vi "Initialize Scanning Task.vi"(0 "NI Force Task in":refnum<class "NI Force Task.lvclass">, 1 "Pot Calibration Cluster":cluster{"Left":dbl, "Right":dbl}, 2 "TDMS File":refnum<k34>, 3 "EMG info":cluster{"Collect EMG?":bool, "EMG Rate":u16}, 4 "DAQ  Channels In":T1={"Force Transducer: Left"="Dev1/ai6", "Force Transducer: Right "="Dev1/ai8", "EMG: Left"="", "EMG: Right"="", "Potentiometer: Left"="", "Potentiometer: Right"=""}, 5 "error in (no error)":errorcluster, 7 "Task Info In":T2={"Number of Trials"=1, "Sampling Rate (Hz)"=200, "Trial Duration (s)"=10, "Adjusted MVC (N)"=5.0, "R Phase"=0, "L Phase"=0, "L Pattern"=1, "R Pattern"=1, "Time Between Trials (s)"=5, "Lissajous Speed"=200} {"Lissajous Speed" min=1 max=200; "Time Between Trials (s)" min=1 step=1; "R Pattern" min=1 max=20 step=1; "L Pattern" min=1 max=20 step=1; "L Phase" max=360 step=1; "R Phase" max=360 step=1; "Adjusted MVC (N)" min=1.0 step=1.0; "Trial Duration (s)" min=1 step=1; "Sampling Rate (Hz)" min=1 step=1; "Number of Trials" min=1 step=1}) -> (14 "NI Force Task out":refnum<class "NI Force Task.lvclass">, 19 "error out":errorcluster)   [LabVIEW 2020, in "NI Force Task.lvlib" / "NI Force Task.lvclass"]
uses:
  NI Force Task.lvclass
  Task info df.ctl
  NI Force Task.lvclass/NI Force Task.ctl
  <vilib>/DAQmx/create/channels.llb/DAQmx Create Channel (AI-Voltage-Basic).vi
  <vilib>/DAQmx/configure/timing.llb/DAQmx Timing (Sample Clock).vi
panel:
  out "error out 2":errorcluster
  # "Left Arm"
  # "Right Arm"
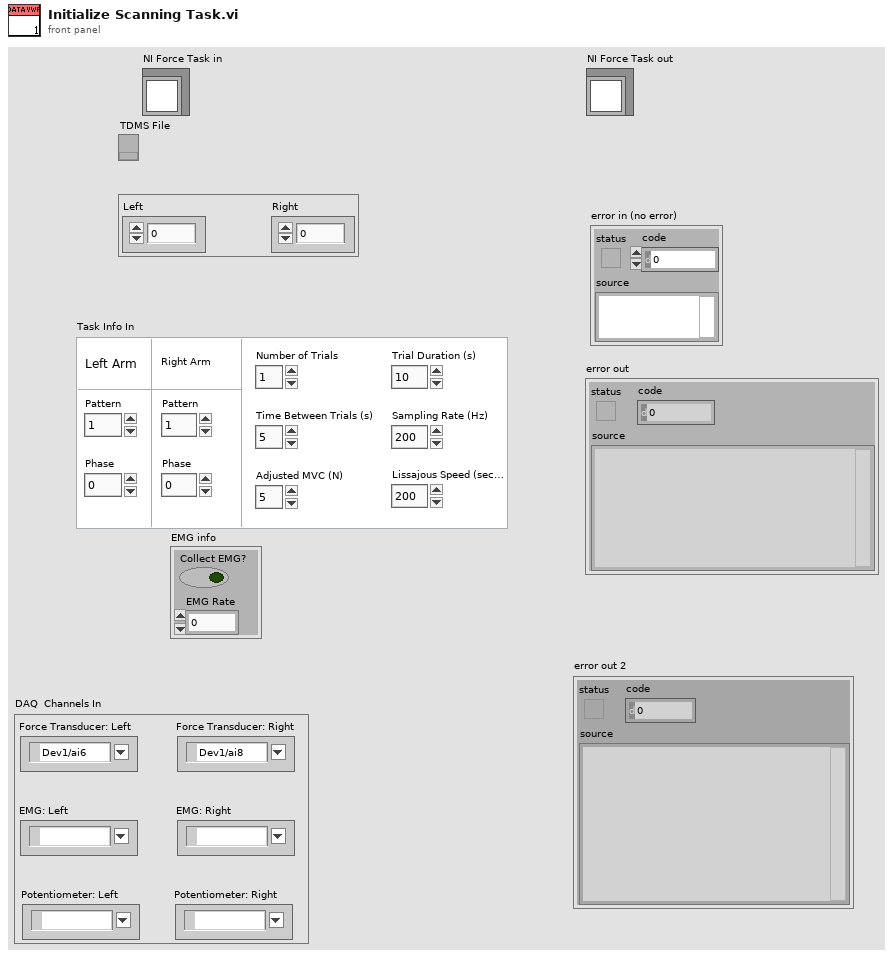
[diagram p1: front panel]
types:
  T1 = cluster{"Force Transducer: Left":tag, "Force Transducer: Right ":tag, "EMG: Left":tag, "EMG: Right":tag, "Potentiometer: Left":tag, "Potentiometer: Right":tag}
  T2 = typedef "Task info df.ctl" = cluster{"Number of Trials":u8, "Sampling Rate (Hz)":u16, "Trial Duration (s)":u8, "Adjusted MVC (N)":dbl, "R Phase":i32, "L Phase":i32, "L Pattern":u8, "R Pattern":u8, "Time Between Trials (s)":u8, "Lissajous Speed":u16}
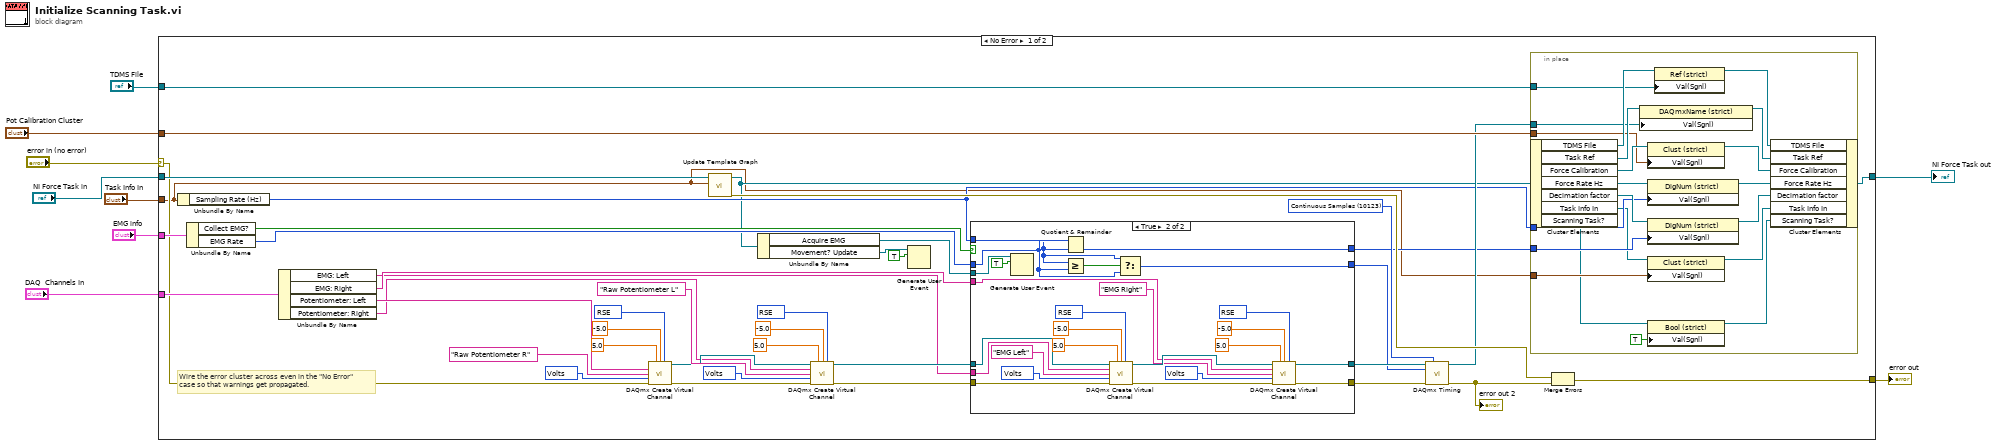
[diagram p0: block diagram]
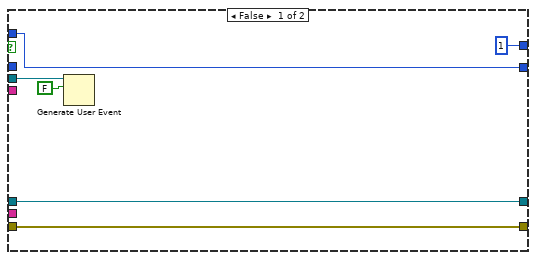
[diagram p2: hidden frame]
diagram:
  n1 = case shown="No Error" "error in (no error)" {
    selector: "error in (no error)" -> [w27 w105]
    tunnel: [w24 w105] -> w8
    tunnel: [w23 w104] -> w6
    tunnel: "NI Force Task in" -> [w51 w104]
    tunnel: "Task Info In" -> [w10 _]
    tunnel: "EMG info" -> [w50 _]
    tunnel: "DAQ  Channels In" -> [w48 _]
    tunnel: "Pot Calibration Cluster" -> [w22 _]
    tunnel: "TDMS File" -> [w20 _]
    frame No Error {
      w28 = 10123 items=["Finite Samples"=10178, "Continuous Samples"=10123, "Hardware Timed Single Point"=12522] ("sample mode")
      w38 = 10348 items=["Volts"=10348, "From Custom Scale"=10065] ("units")
      w42 = 10083 items=["Default"=-1, "RSE"=10083, "NRSE"=10078, "Differential"=10106, "Pseudodifferential"=12529] ("input terminal configuration")
      w43 = 10348 items=["Volts"=10348, "From Custom Scale"=10065] ("units")
      w47 = 10083 items=["Default"=-1, "RSE"=10083, "NRSE"=10078, "Differential"=10106, "Pseudodifferential"=12529] ("input terminal configuration")
      # "Wire the error cluster across even in the \"No Error\"\ncase so that warnings get propagated."
      n2 = Unbundle By Name(w10) -> ("Sampling Rate (Hz)"=w15:u16)
      n3 = Unbundle By Name(w50) -> ("Collect EMG?"=w49:bool, "EMG Rate"=w29:u16)
      n4 = Unbundle By Name(w48) -> ("EMG: Left"=w17:tag, "EMG: Right"=w18:tag, "Potentiometer: Left"=w35:tag, "Potentiometer: Right"=w34:tag)
      n5 = call-poly <vilib>:"DAQmx Create Virtual Channel.vi"("maximum value"=5.0, "minimum value"=-5.0, "input terminal configuration"=w47, "physical channels"=w35, "name to assign"="Raw Potentiometer R", "units"=w43, "error in"=w27) -> ("task out"=w37:refnum<k21>, "error out"=w36:errorcluster)  [unwired: 7 in]
      n6 = call "Update Template Graph.vi"("Task Info In"=w10, "NI Force Task in"=w51) -> ("error out"=w26:errorcluster, "NI Force Task out"=w14:refnum<class "NI Force Task.lvclass">)  [unwired: 8 in]
      n7 = Unbundle By Name(w14) -> ("Acquire EMG"=w13:refnum<user-event>, "Movement? Update"=w12:refnum<user-event>)
      n8 = call-poly <vilib>:"DAQmx Create Virtual Channel.vi"("task in"=w37, "maximum value"=5.0, "minimum value"=-5.0, "input terminal configuration"=w42, "physical channels"=w34, "name to assign"="Raw Potentiometer L", "units"=w38, "error in"=w36) -> ("task out"=w33:refnum<k21>, "error out"=w32:errorcluster)  [unwired: 6 in]
      n9 = Generate User Event(user event=w12, event data cluster=TRUE ("event data")) -> ()  [unwired: 2 in, 2 out]
      n10 = case shown="True" w49 {
        tunnel: w33 -> [w57 w72]
        tunnel: [w57 w64] -> w31
        tunnel: [w56 w63] -> w30
        tunnel: w32 -> [w56 w71]
        tunnel: w15 -> [w55 w61]
        tunnel: w29 -> [_ w62]
        tunnel: [w55 w81] -> w19
        tunnel: w18 -> [_ w66]
        tunnel: w17 -> [_ w65]
        tunnel: [u16 1 w60] -> w16
        tunnel: w13 -> [w53 w59]
        frame False {
          n11 = Generate User Event(user event=w53, event data cluster=FALSE ("event data")) -> ()  [unwired: 2 in, 2 out]
        }
        frame True {
          w73 = 10348 items=["Volts"=10348, "From Custom Scale"=10065] ("units")
          w76 = 10083 items=["Default"=-1, "RSE"=10083, "NRSE"=10078, "Differential"=10106, "Pseudodifferential"=12529] ("input terminal configuration")
          w77 = 10348 items=["Volts"=10348, "From Custom Scale"=10065] ("units")
          w80 = 10083 items=["Default"=-1, "RSE"=10083, "NRSE"=10078, "Differential"=10106, "Pseudodifferential"=12529] ("input terminal configuration")
          n12 = Generate User Event(user event=w59, event data cluster=TRUE ("event data")) -> ()  [unwired: 2 in, 2 out]
          n13 = Greater Or Equal?(x=w61, y=w62) -> (x >= y?=w82:bool)
          n14 = Quotient & Remainder(x=w62, y=w61) -> (floor(x/y)=w60:u16)  [unwired: 1 out]
          n15 = call-poly <vilib>:"DAQmx Create Virtual Channel.vi"("task in"=w72, "maximum value"=5.0, "minimum value"=-5.0, "input terminal configuration"=w80, "physical channels"=w65, "name to assign"="EMG Left", "units"=w77, "error in"=w71) -> ("task out"=w70:refnum<k21>, "error out"=w69:errorcluster)  [unwired: 6 in]
          n16 = Select(t=w61, s=w82, f=w62) -> (s? t:f=w81:u16)
          n17 = call-poly <vilib>:"DAQmx Create Virtual Channel.vi"("task in"=w70, "maximum value"=5.0, "minimum value"=-5.0, "input terminal configuration"=w76, "physical channels"=w66, "name to assign"="EMG Right", "units"=w73, "error in"=w69) -> ("task out"=w64:refnum<k21>, "error out"=w63:errorcluster)  [unwired: 6 in]
        }
      }
      n18 = call-poly <vilib>:"DAQmx Timing.vi"("task/channels in"=w31, "sample mode"=w28, "rate"=w19, "error in"=w30) -> ("task out"=w21:refnum<k21>, "error out"=w25:errorcluster)  [unwired: 10 in]
      "error out 2" <- w25
      n19 = in-place {
        in-place-border: w22 -> [w95]
        in-place-border: w21 -> [w101]
        in-place-border: w20 -> [w100]
        in-place-border: w16 -> [w90]
        in-place-border: w15 -> [w89]
        in-place-border: w10 -> [w86]
        n20 = in-place-cluster #1(w14) -> ("TDMS File"=w103:refnum<vi>, "Task Ref"=w102:refnum<vi>, "Force Calibration"=w97:refnum<vi>, "Force Rate Hz"=w94:refnum<vi>, "Decimation factor"=w92:refnum<vi>, "Task Info In"=w88:refnum<vi>, "Scanning Task?"=w85:refnum<vi>)
        n21 = property class="DAQmxName (strict)"(reference=w102, "Val(Sgnl)"=w101) -> (reference out=w98:refnum<vi>)  [unwired: 1 in, 1 out]
        n22 = property class="Clust (strict)"(reference=w97, "Val(Sgnl)"=w95) -> (reference out=w96:refnum<vi>)  [unwired: 1 in, 1 out]
        n23 = property class="DigNum (strict)"(reference=w94, "Val(Sgnl)"=w89) -> (reference out=w93:refnum<vi>)  [unwired: 1 in, 1 out]
        n24 = property class="DigNum (strict)"(reference=w92, "Val(Sgnl)"=w90) -> (reference out=w91:refnum<vi>)  [unwired: 1 in, 1 out]
        n25 = property class="Clust (strict)"(reference=w88, "Val(Sgnl)"=w86) -> (reference out=w87:refnum<vi>)  [unwired: 1 in, 1 out]
        n26 = property class="Bool (strict)"(reference=w85, "Val(Sgnl)"=TRUE ("Value (Signaling)")) -> (reference out=w84:refnum<vi>)  [unwired: 1 in, 1 out]
        n27 = property class="Ref (strict)"(reference=w103, "Val(Sgnl)"=w100) -> (reference out=w99:refnum<vi>)  [unwired: 1 in, 1 out]
        n28 = in-place-cluster #1("TDMS File"=w99, "Task Ref"=w98, "Force Calibration"=w96, "Force Rate Hz"=w93, "Decimation factor"=w91, "Task Info In"=w87, "Scanning Task?"=w84) -> (w23:refnum<class "NI Force Task.lvclass">)
      }
      n29 = Merge Errors(w26, w25) -> (w24:errorcluster)
    }
    frame Error {
    }
  }
  "error out" <- w8
  "NI Force Task out" <- w6
